vi "cRIO Module Info.vi"(8 "error in (no error)":errorcluster, 9 "session":refnum<k21>="localhost", 10 "number of slots":i32, 11 "cRIO Backplane":T1) -> (0 "error out":errorcluster, 2 "cRIO Modules":T1[](array[typedef]))   [LabVIEW 2017, in "cRIODetectHW.lvlib"]
doc: "Gets information about cRIO modules, such as module ID, vendor name, model name, and serial number."
uses:
  <vilib>/addons/cRIODetectHW/cRIODetectHW.lvlib
  <vilib>/addons/cRIODetectHW/control/cRIO Product Info.ctl
  <vilib>/addons/cRIODetectHW/control/FPGARef.ctl
  <vilib>/nisyscfg/Close (Hardware).vi
  <vilib>/Utility/error.llb/Error Cluster From Error Code.vi
  <vilib>/rvi/errors/niLvFpgaAdjustHostInterfaceError.vi
  <vilib>/FPGAPlugInAG/Dynamic/niLvFpga_Close_Dynamic.vi
  <vilib>/rvi/interface/nirviReadWriteControl/nirviReadWriteControl.xnode
  <vilib>/rvi/interface/nirviCloseFPGA/nirviCloseFPGA.xnode
  NiFpgaLv.dll
  <vilib>/rvi/interface/Simulation/niFpgaSimulationCallBeginRW.vi
  <vilib>/nisyscfg/nisyscfg.lvlib
  <resource>/objmgr/motionsysapi.rc
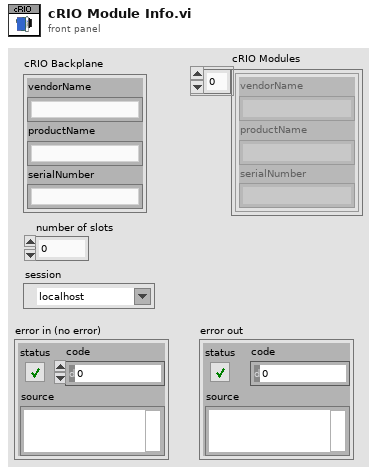
[diagram p1: front panel]
types:
  T1 = typedef "cRIODetectHW.lvlib/cRIO Product Info.ctl" = cluster{"vendorName":string, "productName":string, "serialNumber":string}
  T2 = typedef "cRIODetectHW.lvlib/FPGARef.ctl" = refnum<k20>
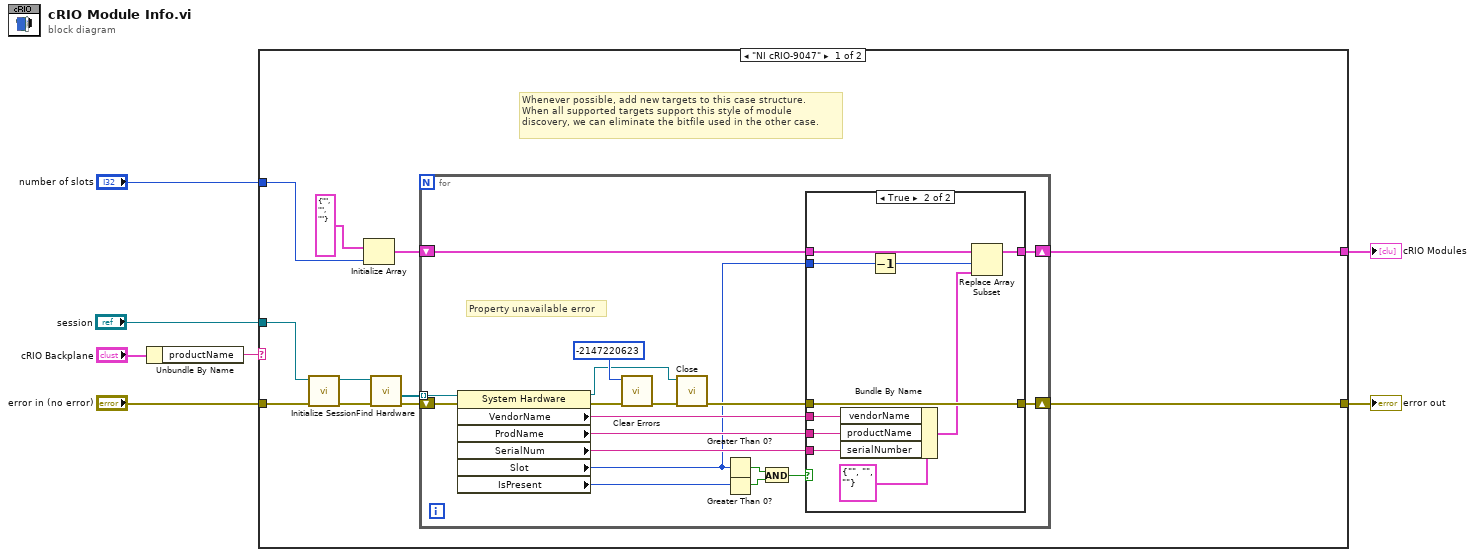
[diagram p0: block diagram]
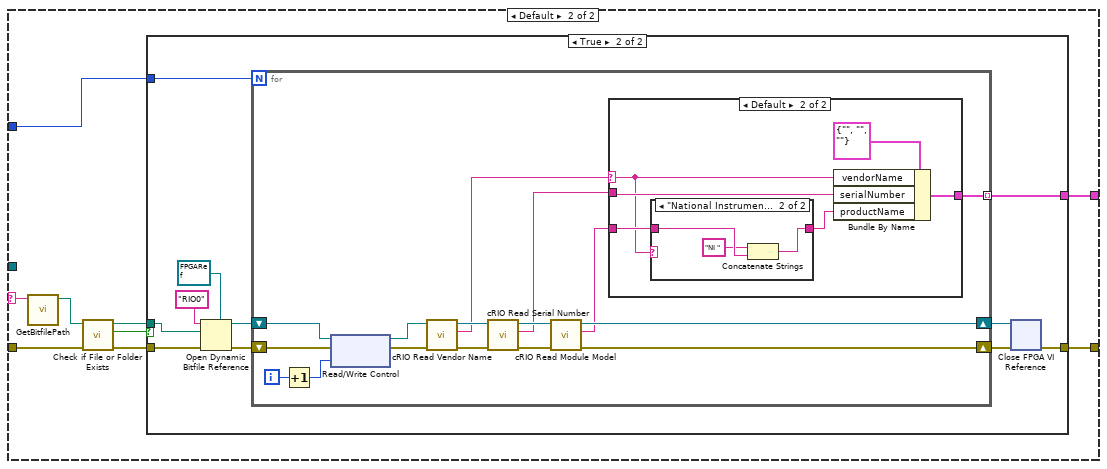
[diagram p3: hidden frame]
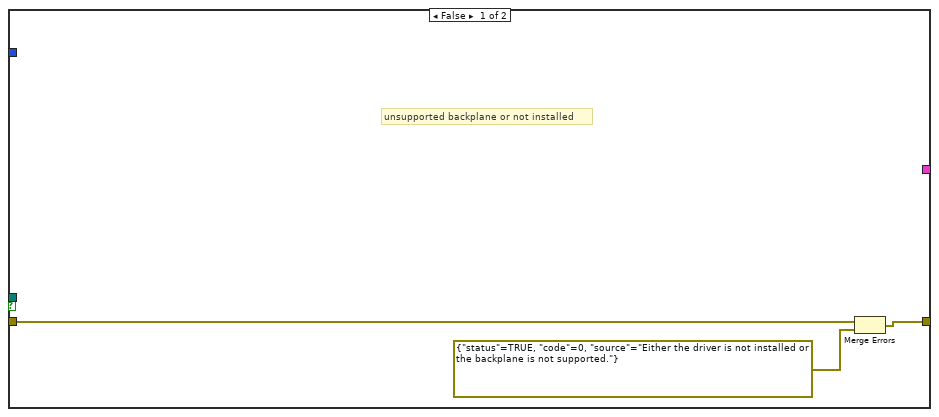
[diagram p4: hidden frame]
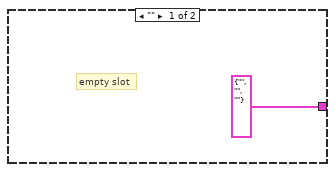
[diagram p5: hidden frame]
diagram:
  n1 = Unbundle By Name("cRIO Backplane") -> ("productName"=w2:string)
  n2 = case shown="\"NI cRIO-9047\"" w2 {
    selector: w2 -> [_ w49]
    tunnel: [w8 w57] -> w7
    tunnel: "number of slots" -> [w11 w56]
    tunnel: "error in (no error)" -> [w15 w55]
    tunnel: [w9 w50] -> w4
    tunnel: "session" -> [w16 _]
    frame "NI cRIO-9047" {
      # "Whenever possible, add new targets to this case structure.\nWhen all supported targets support this style of module\ndiscovery, we can eliminate the bitfile used in the other case."
      n3 = call <vilib>:"Initialize Session.vi"("error in (no error)"=w15, "Target (localhost)"=w16) -> ("error out"=w17:errorcluster, "Session out"=w18:refnum<k21>)  [unwired: 8 in]
      n4 = Initialize Array(T1 {"vendorName"="", "productName"="", "serialNumber"=""} ("cRIO Module Info"), w11) -> (w10:T1[])
      n5 = call <vilib>:"Find Hardware.vi"("error in (no error)"=w17, "Session in"=w18) -> ("error out"=w14:errorcluster, "Resources out"=w13:refnum<k20>[])  [unwired: 6 in, 2 out]
      n6 = for {
        shift-right: [w22] -> w8
        shift-left: w14 -> [w36]
        tunnel: w13 -> [w35] mode=indexing
        shift-right: [w21] -> w9
        shift-left: w10 -> [w20]
        # "Property unavailable error"
        n7 = property class="System Hardware"(reference=w35, error in=w36) -> (reference out=w32:refnum<k20>, error out=w33:errorcluster, "VendorName"=w25:string, "ProdName"=w24:string, "SerialNum"=w23:string, "Slot"=w19:i32, "IsPresent"=w29:i32)
        n8 = call <vilib>:"Clear Errors.vi"("error in (no error)"=w33, "specific error code to clear (0: all)"=-2147220623) -> ("error out"=w31:errorcluster)  [unwired: 4 in, 1 out]
        n9 = call-poly <vilib>:"Close.vi"("error in (no error)"=w31, "Resource in"=w32) -> ("error out"=w30:errorcluster)  [unwired: 9 in]
        n10 = Greater Than 0?(x=w19) -> (x > 0?=w27:bool)
        n11 = Greater Than 0?(x=w29) -> (x > 0?=w28:bool)
        n12 = And(x=w27, y=w28) -> (x .and. y?=w26:bool)
        n13 = case shown="True" w26 {
          tunnel: w30 -> [w38 w44]
          tunnel: w25 -> [_ w47]
          tunnel: w24 -> [_ w46]
          tunnel: w23 -> [_ w45]
          tunnel: [w38 w44] -> w22
          tunnel: [w37 w42] -> w21
          tunnel: w20 -> [w37 w43]
          tunnel: w19 -> [_ w39]
          frame False {
          }
          frame True {
            n14 = Bundle By Name(cluster=T1 {"vendorName"="", "productName"="", "serialNumber"=""} ("cRIO Module Info"), "vendorName"=w47, "productName"=w46, "serialNumber"=w45) -> (w41:T1)
            n15 = Decrement(x=w39) -> (x-1=w40:i32)
            n16 = Replace Array Subset(array=w43, new element=w41, index=w40) -> (w42:T1[])
          }
        }
      }
    }
    frame Default {
      n17 = call <vilib>:"GetBitfilePath.vi"("productName"=w49) -> ("bitfile path"=w54:path)  [unwired: 10 in]
      n18 = call <vilib>:"Check if File or Folder Exists.vi"("error in (no error)"=w55, "path"=w54) -> ("error out"=w53:errorcluster, "file or folder exists?"=w51:bool, "dup path"=w52:path)  [unwired: 7 in]
      n19 = case shown="True" w51 {
        tunnel: [w60 w70] -> w57
        tunnel: [_ w69] -> w50
        tunnel: w56 -> [_ w68]
        tunnel: w53 -> [w58 w67]
        tunnel: w52 -> [_ w61]
        frame False {
          # "unsupported backplane or not installed"
          n20 = Merge Errors(w58, errorcluster {"status"=TRUE, "code"=0, "source"="Either the driver is not installed or the backplane is not supported."} ("error out")) -> (w60:errorcluster)
        }
        frame True {
          n21 = Open Dynamic Bitfile Reference(0:"RIO0" ("Device address"), 1:w61, 3:w67, 4:T2 refnum ("FPGA VI Reference")) -> (5:w66:T2, 8:w65:errorcluster)  [unwired: 1 in]
          n22 = for {
            N: w68 -> [_]
            tunnel: [w78] -> w69 mode=indexing
            shift-right: [w86] -> w64
            shift-left: w65 -> [w75]
            shift-right: [w87] -> w71
            shift-left: w66 -> [w74]
            i -> [w73]
            n23 = Increment(x=w73) -> (x+1=w72:i32)
            n24 = xnode "Read/Write Control"("FPGA VI Reference In"=w74, "error in"=w75, "Module"=w72) -> ("FPGA VI Reference Out"=w80:T2, "error out"=w81:errorcluster)
            n25 = call <vilib>:"cRIO Read Vendor Name.vi"("error in (no error)"=w81, "Refnum in"=w80) -> ("error out"=w82:errorcluster, "Vendor Name"=w77:string, "Refnum out"=w83:T2)  [unwired: 7 in]
            n26 = call <vilib>:"cRIO Read Serial Number.vi"("error in (no error)"=w82, "Refnum in"=w83) -> ("error out"=w85:errorcluster, "Serial Number"=w76:string, "Refnum out"=w84:T2)  [unwired: 7 in]
            n27 = call <vilib>:"cRIO Read Module Model.vi"("error in (no error)"=w85, "Refnum in"=w84) -> ("error out"=w86:errorcluster, "Module Model"=w79:string, "Refnum out"=w87:T2)  [unwired: 7 in]
            n28 = case shown="Default" w77 {
              selector: w77 -> [_ w89]
              tunnel: w79 -> [_ w92]
              tunnel: [T1 {"vendorName"="", "productName"="", "serialNumber"=""} ("cRIO Module Info") w94] -> w78
              tunnel: w76 -> [_ w90]
              frame "" {
                # "empty slot"
              }
              frame Default {
                n29 = case shown="\"National Instruments\"" w89 {
                  tunnel: w92 -> [w95 w98]
                  tunnel: [w95 w97] -> w91
                  frame Default {
                  }
                  frame "National Instruments" {
                    n30 = Concatenate Strings("NI " ("string"), w98) -> (w97:string)
                  }
                }
                n31 = Bundle By Name(cluster=T1 {"vendorName"="", "productName"="", "serialNumber"=""} ("cRIO Module Info"), "vendorName"=w89, "serialNumber"=w90, "productName"=w91) -> (w94:T1)
              }
            }
          }
          n32 = xnode "Close FPGA VI Reference"("FPGA VI Reference In"=w71, "error in"=w64) -> ("error out"=w70:errorcluster)
        }
      }
    }
  }
  "error out" <- w7
  "cRIO Modules" <- w4
